vi "Puzzle 1-2.vi"() -> ()   [LabVIEW 2022 SP3]
panel:
  out "sum":i32=54265
  out "Array 3":i32[](array[numeric])=[91, 57, 81, 79, 28, 41, 41, 27, 45, 61, 17, 82, 27, 72, 45, 76, 32, 22, 13, 88, 15, 67, 85, 75, 55, 25, 75, 76, 72, 41, 58, 51, 13, 82, 73, 22, 73, 86, 32, 71, 92, 15, 49, 91, 17, 18, 32, 99, 77, 92, 38, 53, 25, 97, 22, 28, 84, 65, 28, 94, 47, 68, 63, 36, 66, 71, 51, 35, 91, 54, 43, 44, 18, 71, 96, 21, 37, 17, 27, 86, 38, 96, 16, 23, 51, 44, 72, 55, 71, 97, 82, 79, 99, 62, 88, 11, 88, 71, 65, 42, 61, 53, 33, 61, 39, 23, 24, 96, 24, 19, 65, 48, 11, 79, 38, 13, 13, 48, 21, 77, 55, 39, 32, 22, 16, 22, 64, 95, 96, 43, 29, 71, 22, 89, 29, 18, 91, 98, 43, 65, 11, 74, 63, 11, 74, 56, 41, 82, 38, 18, 71, 64, 96, 19, 81, 99, 13, 88, 95, 43, 15, 33, 46, 22, 87, 52, 29, 69, 92, 11, 17, 11, 96, 22, 96, 34, 32, 54, 43, 79, 56, 88, 51, 91, 71, 91, 37, 35, 66, 87, 71, 16, 14, 25, 16, 66, 98, 29, 31, 98, 87, 33, 18, 63, 62, 11, 88, 56, 66, 92, 18, 26, 94, 62, 58, 42, 19, 41, 64, 61, 52, 17, 92, 38, 79, 19, 95, 32, 35, 15, 96, 89, 67, 57, 53, 13, 36, 48, 89, 38, 71, 55, 55, 21, 85, 17, 55, 23, 28, 87, 77, 34, 39, 92, 19, 94, 72, 27, 37, 21, 22, 73, 57, 29, 42, 73, 64, 85, 64, 21, 72, 31, 54, 82, 65, 11, 22, 53, 28, 12, 94, 12, 62, 96, 47, 31, 74, 37, 33, 84, 42, 77, 28, 17, 34, 47, 42, 87, 36, 74, 98, 38, 49, 26, 28, 14, 23, 59, 88, 11, 15, 45, 85, 53, 19, 37, 86, 14, 52, 64, 48, 85, 71, 79, 11, 11, 79, 89, 89, 31, 56, 48, 95, 75, 63, 72, 89, 88, 58, 78, 47, 42, 15, 48, 77, 36, 85, 68, 93, 73, 52, 82, 58, 34, 22, 12, 86, 35, 91, 19, 13, 44, 95, 52, 58, 51, 65, 13, 61, 13, 87, 69, 63, 45, 24, 47, 42, 49, 28, 61, 21, 33, 99, 27, 65, 24, 74, 73, 74, 72, 29, 87, 94, 29, 88, 53, 24, 77, 45, 33, 64, 89, 16, 68, 92, 36, 98, 16, 78, 53, 27, 26, 34, 47, 88, 49, 23, 52, 88, 91, 99, 87, 62, 66, 88, 67, 57, 59, 61, 48, 69, 57, 55, 99, 22, 26, 45, 17, 63, 38, 74, 23, 17, 93, 63, 23, 91, 94, 54, 67, 55, 89, 57, 67, 89, 79, 29, 31, 48, 73, 48, 29, 17, 51, 44, 82, 72, 53, 12, 21, 11, 33, 56, 61, 53, 32, 98, 59, 66, 86, 46, 14, 89, 14, 11, 29, 79, 95, 67, 76, 88, 99, 42, 49, 53, 18, 35, 19, 33, 75, 64, 77, 24, 97, 41, 83, 94, 23, 99, 15, 24, 61, 72, 63, 44, 72, 13, 25, 64, 43, 28, 44, 37, 27, 53, 91, 95, 75, 66, 61, 38, 38, 54, 87, 96, 71, 29, 25, 81, 13, 11, 58, 74, 38, 32, 96, 35, 88, 34, 63, 75, 61, 41, 11, 11, 91, 39, 56, 77, 77, 77, 23, 87, 89, 17, 47, 55, 98, 52, 27, 91, 98, 87, 67, 35, 35, 15, 78, 19, 85, 17, 41, 23, 52, 97, 19, 68, 39, 43, 44, 27, 12, 86, 23, 87, 28, 49, 83, 92, 62, 72, 24, 23, 56, 18, 58, 32, 17, 11, 15, 77, 33, 84, 47, 73, 95, 82, 48, 43, 97, 35, 12, 13, 95, 27, 57, 67, 34, 88, 33, 99, 39, 97, 33, 62, 76, 63, 14, 84, 71, 52, 21, 37, 93, 48, 57, 29, 73, 14, 68, 19, 33, 97, 29, 86, 22, 92, 64, 42, 27, 66, 62, 22, 43, 68, 82, 44, 95, 74, 75, 37, 15, 89, 81, 43, 61, 53, 34, 45, 86, 31, 55, 43, 92, 88, 94, 87, 54, 41, 34, 45, 22, 63, 44, 23, 47, 54, 97, 18, 14, 77, 36, 48, 89, 49, 97, 71, 73, 41, 83, 91, 48, 89, 39, 97, 88, 28, 73, 61, 11, 62, 12, 24, 76, 22, 96, 18, 95, 56, 55, 17, 98, 61, 78, 73, 45, 94, 16, 65, 15, 88, 62, 57, 55, 91, 28, 99, 31, 61, 27, 79, 34, 64, 99, 42, 22, 13, 66, 37, 28, 22, 45, 65, 36, 77, 84, 14, 11, 29, 64, 97, 45, 96, 65, 18, 84, 29, 87, 32, 75, 89, 33, 17, 11, 39, 56, 79, 42, 75, 49, 72, 93, 39, 58, 16, 19, 36, 65, 44, 64, 52, 24, 16, 38, 74, 59, 38, 56, 65, 73, 72, 24, 27, 23, 11, 26, 82, 92, 82, 88, 79, 98, 44, 78, 91, 35, 14, 59, 58, 77, 98, 95, 95, 51, 15, 64, 46, 64, 38, 24, 85, 59, 17, 15, 62, 95, 22, 88, 14, 12, 52, 82, 22, 52, 83, 46, 55, 52, 22, 83, 54, 68, 53, 31, 26, 55, 35, 38, 58, 24, 33, 85, 81, 95, 32, 83, 54, 71, 71, 65, 45, 74, 96, 88, 33, 39, 14, 14, 71, 96, 43, 18, 56, 16, 66, 79, 23, 15, 54, 17, 85, 97, 23, 65, 94, 97, 59, 24, 66, 49, 31, 19, 19, 49, 66, 82, 75, 18, 86, 66, 98, 24, 44, 63, 63, 46, 33, 36, 97, 24, 47, 83, 74, 52, 95, 83, 52, 74, 11, 54, 49, 63, 88, 71, 54, 29, 55, 98, 56, 31, 48, 32, 71, 68, 11, 69, 86, 96, 49, 25, 33, 51, 91, 52, 48, 34, 37, 55, 48, 81, 48, 43, 69, 44, 49, 64, 94, 67, 99, 58, 86, 72, 78, 87, 46, 53, 27, 66, 89, 51, 42, 68, 47, 32, 57, 43, 72, 97, 87, 29]
  out "Array 2":string[](array[string])=["nine", "5", "8", "7", "2", "four", "four", "2", "4", "6", "1", "eight", "two", "seven", "4", "7", "3", "2", "1", "8", "1", "6", "eight", "7", "5", "two", "7", "7", "7", "4", "5", "five", "one", "8", "7", "2", "7", "8", "three", "7", "9", "1", "four", "nine", "1", "one", "three", "9", "7", "nine", "3", "5", "two", "nine", "2", "2", "eight", "six", "2", "nine", "four", "6", "six", "3", "6", "seven", "five", "3", "9", "5", "four", "4", "1", "seven", "9", "2", "three", "1", "2", "8", "three", "nine", "1", "2", "5", "4", "seven", "5", "7", "9", "8", "7", "9", "6", "eight", "1", "8", "seven", "six", "4", "6", "5", "3", "six", "3", "two", "two", "nine", "2", "one", "6", "4", "1", "7", "three", "1", "1", "4", "two", "7", "5", "three", "3", "2", "1", "2", "six", "nine", "9", "four", "two", "7", "2", "8", "2", "one", "nine", "9", "4", "6", "1", "seven", "six", "one", "7", "5", "4", "eight", "3", "1", "seven", "six", "nine", "one", "8", "9", "one", "eight", "nine", "four", "one", "3", "four", "2", "8", "five", "2", "6", "nine", "one", "one", "1", "nine", "2", "nine", "three", "3", "5", "4", "7", "5", "eight", "5", "nine", "seven", "nine", "three", "3", "six", "eight", "seven", "1", "one", "2", "one", "6", "nine", "two", "3", "9", "8", "3", "1", "6", "6", "one", "8", "five", "6", "nine", "1", "2", "9", "6", "5", "four", "1", "4", "6", "6", "five", "one", "9", "3", "7", "one", "9", "three", "3", "one", "nine", "8", "six", "five", "five", "1", "three", "4", "eight", "3", "7", "5", "five", "two", "eight", "one", "five", "two", "two", "8", "seven", "3", "3", "9", "one", "9", "seven", "two", "three", "2", "2", "seven", "5", "two", "4", "seven", "six", "8", "6", "2", "seven", "three", "5", "8", "six", "1", "two", "5", "2", "one", "9", "one", "six", "nine", "4", "3", "seven", "3", "3", "eight", "4", "seven", "2", "1", "three", "four", "four", "eight", "three", "7", "9", "3", "4", "two", "two", "one", "2", "five", "eight", "1", "one", "four", "8", "five", "1", "3", "8", "1", "5", "6", "four", "8", "7", "7", "1", "one", "seven", "8", "8", "3", "5", "4", "nine", "seven", "6", "seven", "eight", "8", "5", "7", "four", "four", "1", "4", "7", "three", "8", "six", "9", "seven", "five", "eight", "five", "three", "2", "one", "8", "three", "9", "one", "one", "four", "9", "five", "five", "5", "six", "1", "6", "one", "eight", "six", "6", "four", "2", "four", "4", "4", "two", "6", "two", "three", "9", "2", "six", "2", "seven", "7", "seven", "7", "two", "8", "nine", "two", "eight", "five", "2", "7", "four", "3", "six", "8", "one", "six", "9", "3", "9", "one", "seven", "5", "2", "2", "three", "4", "8", "four", "two", "5", "eight", "nine", "9", "eight", "six", "6", "eight", "6", "5", "five", "6", "four", "6", "5", "5", "9", "two", "two", "4", "1", "six", "three", "7", "2", "1", "9", "six", "2", "nine", "9", "five", "6", "five", "eight", "5", "six", "8", "7", "two", "3", "4", "seven", "four", "2", "1", "5", "four", "8", "7", "5", "1", "2", "one", "3", "five", "six", "5", "three", "9", "5", "6", "eight", "4", "1", "eight", "one", "one", "2", "seven", "9", "6", "7", "eight", "9", "four", "4", "5", "1", "3", "one", "3", "seven", "six", "7", "2", "9", "4", "eight", "9", "two", "9", "one", "2", "six", "7", "6", "4", "7", "1", "two", "six", "4", "2", "4", "three", "two", "five", "nine", "9", "7", "6", "six", "three", "three", "5", "8", "nine", "7", "two", "2", "8", "1", "1", "five", "seven", "three", "three", "nine", "3", "8", "3", "six", "seven", "6", "4", "one", "one", "nine", "3", "five", "7", "7", "7", "2", "8", "8", "one", "four", "5", "9", "5", "2", "nine", "9", "8", "6", "3", "3", "1", "seven", "1", "eight", "1", "4", "2", "5", "nine", "one", "6", "3", "4", "four", "two", "one", "eight", "2", "8", "2", "4", "eight", "nine", "six", "7", "two", "two", "5", "1", "5", "three", "1", "1", "1", "7", "3", "8", "four", "7", "9", "8", "4", "4", "nine", "3", "one", "one", "9", "two", "5", "6", "three", "8", "3", "9", "3", "nine", "three", "6", "7", "6", "one", "8", "seven", "5", "two", "three", "9", "4", "five", "two", "7", "one", "6", "1", "3", "9", "2", "8", "2", "9", "six", "four", "two", "6", "6", "2", "four", "6", "8", "4", "nine", "seven", "seven", "3", "1", "eight", "eight", "4", "6", "5", "3", "4", "8", "3", "5", "4", "9", "8", "9", "8", "5", "4", "three", "4", "2", "six", "4", "2", "4", "5", "9", "1", "one", "7", "3", "4", "8", "four", "9", "7", "7", "4", "8", "nine", "four", "eight", "three", "nine", "eight", "two", "7", "six", "1", "six", "one", "two", "seven", "2", "9", "one", "nine", "5", "5", "one", "9", "6", "7", "seven", "4", "nine", "1", "6", "one", "8", "6", "five", "5", "nine", "2", "9", "3", "6", "2", "7", "3", "6", "9", "4", "2", "one", "6", "3", "two", "2", "4", "6", "three", "seven", "8", "1", "one", "2", "six", "9", "four", "nine", "six", "1", "8", "2", "eight", "three", "seven", "8", "three", "one", "1", "3", "5", "7", "four", "7", "four", "seven", "nine", "3", "five", "1", "one", "3", "six", "4", "6", "5", "two", "one", "3", "seven", "5", "3", "5", "6", "7", "seven", "2", "2", "2", "1", "2", "eight", "nine", "eight", "eight", "seven", "9", "4", "7", "nine", "three", "1", "5", "five", "7", "9", "9", "nine", "five", "1", "six", "four", "6", "3", "two", "eight", "five", "1", "1", "6", "9", "2", "8", "1", "one", "5", "8", "two", "five", "eight", "four", "five", "five", "2", "8", "5", "6", "5", "3", "2", "5", "three", "3", "5", "two", "3", "8", "8", "9", "3", "eight", "five", "7", "seven", "six", "four", "7", "9", "eight", "three", "3", "one", "one", "seven", "9", "4", "one", "5", "one", "six", "7", "two", "one", "5", "1", "8", "nine", "2", "6", "nine", "9", "5", "two", "six", "four", "three", "one", "1", "4", "6", "eight", "7", "one", "8", "6", "nine", "2", "4", "6", "six", "4", "3", "three", "9", "2", "4", "8", "7", "5", "nine", "8", "5", "seven", "1", "5", "four", "six", "8", "seven", "5", "two", "five", "9", "five", "3", "four", "3", "7", "six", "one", "six", "eight", "nine", "4", "two", "3", "five", "9", "five", "four", "three", "three", "5", "4", "eight", "4", "four", "six", "4", "4", "6", "nine", "6", "9", "5", "eight", "seven", "seven", "eight", "4", "5", "two", "six", "eight", "5", "4", "6", "4", "three", "five", "4", "seven", "nine", "eight", "two"]
  out "Array":string[](array[string])=["1", "seven", "1", "9", "eight", "1", "1", "seven", "five", "one", "7", "two", "seven", "two", "5", "6", "2", "2", "3", "eight", "five", "seven", "five", "5", "5", "five", "5", "six", "two", "one", "eight", "1", "three", "two", "three", "two", "3", "6", "2", "1", "two", "5", "nine", "one", "seven", "eight", "two", "nine", "7", "2", "eight", "three", "5", "seven", "2", "eight", "4", "five", "8", "four", "seven", "eight", "three", "six", "6", "one", "one", "five", "1", "four", "3", "4", "eight", "1", "6", "one", "7", "seven", "7", "six", "8", "six", "6", "three", "one", "4", "2", "5", "1", "7", "two", "9", "9", "2", "eight", "1", "8", "one", "five", "two", "one", "3", "3", "1", "nine", "3", "four", "six", "four", "9", "5", "eight", "1", "nine", "8", "3", "3", "eight", "1", "7", "5", "nine", "2", "two", "six", "2", "4", "five", "6", "3", "9", "1", "2", "nine", "9", "8", "one", "8", "3", "5", "1", "4", "three", "one", "4", "six", "1", "two", "8", "eight", "1", "4", "six", "9", "one", "9", "3", "eight", "5", "3", "5", "3", "six", "2", "seven", "2", "9", "9", "two", "one", "seven", "1", "6", "2", "six", "4", "2", "4", "three", "nine", "6", "8", "1", "one", "1", "1", "7", "five", "six", "7", "1", "6", "4", "five", "6", "six", "8", "9", "1", "8", "seven", "3", "eight", "three", "2", "1", "eight", "six", "six", "2", "eight", "six", "4", "2", "8", "2", "9", "1", "four", "1", "two", "7", "2", "8", "nine", "nine", "5", "two", "5", "5", "six", "9", "7", "7", "three", "3", "6", "8", "nine", "eight", "1", "5", "5", "1", "five", "7", "5", "three", "eight", "7", "seven", "4", "nine", "two", "nine", "four", "two", "7", "7", "1", "2", "three", "seven", "nine", "2", "3", "4", "five", "4", "1", "two", "one", "four", "2", "five", "one", "2", "3", "8", "2", "4", "2", "two", "six", "7", "1", "four", "seven", "3", "four", "two", "7", "eight", "seven", "4", "7", "2", "seven", "6", "four", "eight", "eight", "9", "6", "eight", "four", "3", "9", "eight", "1", "5", "5", "5", "three", "nine", "seven", "6", "four", "2", "four", "8", "five", "one", "nine", "1", "one", "9", "9", "nine", "1", "six", "eight", "five", "5", "three", "2", "9", "8", "8", "8", "7", "2", "5", "eight", "7", "6", "5", "8", "3", "three", "2", "2", "eight", "4", "2", "2", "6", "five", "one", "9", "three", "4", "five", "2", "eight", "one", "five", "three", "1", "3", "7", "9", "three", "5", "four", "seven", "two", "9", "eight", "1", "1", "three", "9", "7", "5", "4", "4", "3", "four", "2", "nine", "seven", "4", "nine", "8", "3", "four", "7", "5", "three", "four", "9", "6", "8", "2", "six", "8", "6", "eight", "three", "7", "six", "four", "7", "8", "9", "3", "two", "8", "one", "nine", "7", "2", "6", "eight", "seven", "7", "9", "one", "eight", "nine", "seven", "5", "9", "two", "6", "five", "7", "3", "8", "4", "three", "seven", "3", "3", "3", "1", "four", "4", "seven", "5", "nine", "7", "7", "nine", "9", "9", "one", "eight", "3", "eight", "9", "7", "1", "4", "two", "two", "3", "two", "1", "1", "3", "6", "1", "three", "2", "8", "9", "6", "6", "six", "4", "nine", "4", "1", "9", "9", "five", "seven", "six", "8", "nine", "2", "nine", "3", "eight", "5", "nine", "3", "5", "4", "seven", "4", "7", "one", "3", "4", "3", "9", "five", "4", "one", "2", "3", "4", "2", "three", "5", "four", "three", "8", "4", "7", "7", "3", "one", "5", "5", "6", "one", "eight", "eight", "4", "seven", "6", "one", "9", "5", "1", "three", "1", "8", "4", "eight", "two", "six", "5", "8", "4", "3", "5", "1", "1", "1", "one", "one", "9", "6", "7", "7", "7", "three", "7", "9", "7", "7", "5", "8", "two", "seven", "one", "eight", "7", "seven", "5", "five", "5", "8", "nine", "5", "seven", "one", "3", "2", "seven", "9", "8", "nine", "three", "four", "7", "two", "six", "three", "seven", "eight", "nine", "3", "2", "two", "2", "four", "3", "6", "8", "eight", "two", "seven", "1", "5", "7", "3", "4", "7", "3", "five", "two", "8", "3", "seven", "five", "2", "three", "5", "7", "7", "7", "four", "eight", "3", "9", "nine", "seven", "3", "two", "six", "three", "four", "four", "one", "2", "1", "seven", "three", "8", "seven", "nine", "three", "4", "8", "9", "3", "seven", "9", "six", "2", "2", "4", "two", "7", "six", "two", "2", "3", "8", "two", "4", "5", "4", "five", "7", "5", "nine", "1", "three", "1", "3", "4", "5", "6", "one", "5", "three", "two", "8", "4", "seven", "four", "1", "4", "five", "2", "3", "4", "three", "seven", "4", "7", "8", "4", "seven", "6", "eight", "nine", "9", "seven", "1", "3", "1", "three", "one", "eight", "9", "nine", "seven", "8", "8", "three", "one", "1", "two", "2", "4", "six", "two", "6", "8", "five", "6", "five", "seven", "8", "one", "eight", "three", "5", "4", "6", "5", "five", "eight", "2", "7", "5", "1", "8", "9", "one", "one", "7", "nine", "four", "four", "9", "2", "2", "three", "6", "7", "eight", "2", "five", "five", "six", "seven", "4", "4", "1", "9", "four", "seven", "5", "6", "five", "8", "four", "nine", "seven", "2", "5", "9", "three", "7", "1", "nine", "6", "nine", "2", "five", "nine", "two", "three", "nine", "8", "6", "9", "6", "5", "four", "4", "two", "4", "6", "eight", "4", "9", "8", "6", "five", "three", "two", "4", "7", "three", "1", "6", "2", "2", "2", "8", "9", "eight", "4", "8", "one", "5", "four", "nine", "8", "7", "8", "five", "5", "1", "five", "four", "6", "four", "8", "four", "5", "9", "seven", "5", "two", "5", "2", "eight", "4", "2", "2", "2", "2", "two", "3", "6", "five", "two", "2", "three", "four", "8", "three", "one", "6", "five", "5", "eight", "eight", "four", "3", "5", "1", "5", "2", "three", "four", "1", "one", "five", "5", "4", "six", "8", "3", "9", "four", "four", "one", "6", "three", "8", "six", "6", "6", "nine", "3", "five", "4", "7", "5", "7", "3", "five", "4", "7", "nine", "four", "6", "nine", "one", "9", "nine", "9", "6", "2", "five", "8", "6", "six", "eight", "4", "4", "three", "3", "6", "three", "6", "seven", "four", "seven", "three", "four", "2", "five", "3", "two", "4", "1", "four", "9", "3", "8", "one", "four", "9", "5", "eight", "6", "1", "8", "2", "one", "8", "one", "9", "six", "6", "9", "5", "3", "1", "one", "two", "eight", "four", "7", "5", "eight", "one", "8", "three", "nine", "4", "nine", "four", "four", "7", "9", "8", "6", "two", "eight", "seven", "6", "three", "seven", "6", "9", "1", "2", "eight", "seven", "2", "seven", "3", "2", "7", "7", "9"]
  out "subarray":string[](array[string])=["ninefourone1", "53sevenvvqm", "kscpjfdxp895foureightckjjl1", "72fivebt9ndgq", "28gtbkszmrtmnineoneightmx", "four66jqrbtqcsxjtqjvfjhl1", "four8pzznjbhxlhtz6bhtzdxjlg1", "rgxjrsldrfmzq25szhbldzqhrhbjpkbjlsevenseven", "slkjvk4threesevenznjqmmfive", "61ppgrkmkfhteightone", "1threesix67px", "sxbjdbtlnjrmlzgxneightthreepmqxdxhfk8jfrheightwovp", "twofour2sevenk", "sevenonezknqnkfqbzffjvfivetwo94two", "45xj", "mp7one6eightvhfnmfive6", "fhtctftxm3threefour2b", "2dq7bdmhhs92", "pdnbqlbvtcxgpnfhmsfhzstgm173", "8fourvxkddsrlcvseveneight", "15zqpmsix77hlljgfive", "jzjv6seven", "eight1vbfive", "721sixsdzbqtskbpkqbcmgmlpk5psrhr", "pqxdxcx5", "twozsf2five", "7twosixthree775", "7xtxrch7six", "729twofourlqrxtwo", "qtvbgtclhnk4ninefourseven5one", "jvhngkcdjhnmqghdbqdzqssf5onegzjbbcchboneightn", "five8two14five2nine1", "one3twomddthree", "8nine9two", "7fiveeight9ninesix6fivethree", "254kcd61dc4two", "7sixonetxvthntlngtwobzkbz23", "8sixnine6", "threedqtgmv2skmvcd", "7ptdhpvr1", "lsvmzvzvd9mqxszjmbddkmxzdxsninedmglzlzphtwo", "kgdt12seven4xxtttr5", "nrdtgdftjmfour6fxjninenineblqlthvpcx", "ninezmstcdfchc11onebmmfdfhvdncrhc", "1fiveseven", "oneone26twoeight", "threefivenine98one9twotbbcq", "9cm7ninestc", "jcrbmcjtrlzvz7", "nine8nine22", "3nineoneseveneight", "58four2three", "stwonefourthree9twonine4six5bvxgkxf", "ninechzcz4seven", "2tgzgmtzzpjdqqz", "brsptjppb28qxcxxjbzpeighteight", "eightthree3ninejrft4", "sixqsgkzdjmgpfive4threemxltqdxsfive", "vxfd2q8", "khqhgqlxslkmbrvljcnineeight1gjgcqmnbdczqb8four", "mvbltrgpfourcclxftbb7gcbqcptvgfsevenrdm", "61eight", "six8fourthree6fourseven6three", "jqdfxvhjg3sflkn2sixptxxsqrfml", "6jtxs", "seven99threeone", "five6sevensmbbrjqvdbmkbsqtwonelg", "fdvfsndt32fourgllgfrninebhnzzczfive", "9hxp9srhjhjjvqljhzprcjpqreightzs1", "djldhkkcn55threethreefourflnxnbzhkzmx", "fourfive43chfvjnvjrkpxlgjrfnqbl", "fxjgtj4", "1sevenfour2fiveeight", "seven43rxxeightb1", "9sevensnxkp3lpzxfxnntkxzkrhk7jzhmtvn6", "25one", "threeone7", "1pkfvsxxthreeoneseven", "ztbvfqnpz2xdhgdjmgvfourtworqbxqsh47", "8four7sixninesix", "threedgl88cczqhqxjnc", "nineeightthree4sixfive3sixdqlmscqjk", "16crjsdl", "tgq2sixhc7three", "tzgsqspndt5xnqlthghzfvkkhone", "4fxdqrs64ninex34gd", "seven22", "kghfkrpvnppfncbhhqpt55bjf", "hjhb71bqdrrgsrkqdtsgrxgsscqjmtfzjkzsbp", "lgdnt9threeeighteight97", "pvjhnk83sixncvgmsjltwotdmmpxknhvntfndxr", "7449", "qdfzv9hkprplzkfh", "66three5five4zdsfrcnljqmsxf2", "veightwo27bdbsvseveneightrcqcjxsixeight", "1thvkkk", "8bnxqfsdhzppblzlzbkfsksfscmb", "zseventbdzlmhnnrfive1one", "sixxnmntrmp6srcsqbrqnjfiveeightfive", "4trnzlshnjtwo5twocxrvfssbj", "6two3twonetqt", "55qsnx43", "3three23tpctbkrnqv", "sixqk4cnfdmtltmlhqxtwo41glkhdhgnt", "35fivesevenpfournxzsbbgzthjvlvzrnine", "tworkzgkcvcone53nrvgdvgtc", "two9llkjbkz8pklrsgqqzr2four", "ninecgpbgcnine4tldjqsone4six", "2tfjhtfourfour", "onebhlhdvvqx1sevenmsixsix9", "pjgjt6jkrgshxltfnine8four45", "4vsqfljrfiveqeightnvbdb", "11nfslqvhm", "7crrhqxsfive8ctkzbhqnine", "vrvtglvthreettrkq5bdlrtpx718", "1btbxlthreedtrzgeightnineqczhqm3", "193", "fcbzxqxxjtmn47ffschdrbeight", "twoh1gqkrnm1", "7ninesixpzpsn7", "5kkvzpgqd", "three6nine", "32fdn", "22twoxgvktxpxmbjqtgtbckx", "1hdtftwosix", "2jfc", "six5nvzcgmrscjn5eight4", "nineqhtczsninetwosix4five", "9three6sj", "hntktlbqmldrphqzxkhfour193", "twotwo5259", "v7six1vtlxnpm", "rhsm2", "gprmtxbhlsv8onefournine", "2fsrbtdvft15six1kxpqbnqsxh9", "one5onemxthree8", "nineqbxdbznzktxsmstsntzffour3one", "9blhkhjsgsfgsblzdtqqfour8", "stz4889563cb", "vjrbs6threeptbbmncz7hqhqgfgldtseven5", "vbfs1", "zjqgczjsjpvzvjseven4", "sixfjzbrrhcfqvglxhnsxninedrvtvjbfqjdbrzblkq6three", "one3threegcdldjsrsssixonefiveonechngsl", "7srxv4hsgjqsqfvv1tdngkpjrczkl4", "5scgdglnjbnsix8fivesixtjccvmkfxfnzvhctgpncjc", "4eightfivefive1lgscbj7kpcr1", "eightknfssevenfive6jnpklczrpfeightwol", "37qccxllhzshninebvpc8", "1eightmmcthkhf", "seven8fourqn7tbgqnmzcc1", "sixsevenone4", "clhdvjnqnine9threesix", "onetwoeight9", "81z3threenjsdhnqxvtwonezv", "9hqtsb", "onekgnlbthreeg3", "eightspnrpjb65fivevzfpvjntbg7drbgjccneight", "ninerdlsix7285", "fournineninefive3vbnhmhdvjgdqcm", "njzspqxpxrone7four55", "nfdhlqcpvzrrtsmzhgq3", "fourmfdtnpsfbxkjtgtgx5sixrppsqplqdjvnsixdtqvtdm", "21onesix6sixnine2", "fffsmvtt8fivenineglrqrmktzzseven", "fivefoursevencjxmskrqclz2", "lgk27threefourfsqrbkntbkfourvflgrzhh9", "617hj9", "ninegcxninetwohpfdxrb3tjjjtxtnvtwo", "one1gnftc8onehtsxsmg", "foneight3fsbhdqzr5twojbsdnntwohd9seven", "zkzpfvcxqnbvrg1", "nine36cddqfvrf", "rdjlpfk2pschfsdrpz", "nine994three8six", "three3nvflpftf2eight4", "3nine2", "rxxjdk5354", "hf4eight8qjtcfldnkvtwofivetwothree", "7six3twodhnvmxj1nine", "57seven3six6", "qklbvzfhclfnllhhgeight8xtvld", "5fgzqhkssmkcfour1", "hhvjkdnlffnineeighttwo18twonecs", "sevenbfzrgfm1six1", "nine71cskklxvcbnxtskdbqnpgklrxklcgccxjnssksrlkx", "hmklhhjdthree77", "3vpxclbgkpone3ninesrclfive", "djfqkgjvqpfvdsix5sixtwoeightsix", "eightlt7csvgxpnslk", "sevenfoureightnld2mxtgpbzpthree1", "11sevenglfmsb6", "onetjjnxvssg1four4drxbxpnpv24", "2zdxs9mfnbgfmjln1threefive", "one186ltsbck", "6fsbpb9sixhc", "nine818", "xzqcpcdprsqjbgknkvztwo419q", "39qfdlcnkhg31", "9djnlcrxqxhrcb8mczrxrm", "nmb887525seven", "jhmv3", "zhvdbn1fivem8seven4sixoneighttsn", "6zmmjqmnftclqbcthree", "6cpzeight92", "onepqfhtsevencvlfvnczhb91mmtdprqxmcnine1", "tvqdfxn8eight", "five6fivercgrpbtjgv87jmcndclbk2six", "jgtmrbvl68lpqkpxddqqxvsixfivesix", "nine2nlffgkvmp", "1frdnhssftg4eightgclxsgqtn", "2sixblr94six", "94mlfv", "6vlqtcsmdd47hpfmlc7fiveeight2", "tklxghxv5bzc4hhcdcpmnine8", "four6one1zzgqghvs412", "xghjpblsfpg19ntpfmcfd", "471rbdblzs", "69fourhjxkvd7fourfour", "jmrscfqdfppfdjskpk61", "five5eightnqpd9ninezknztwo", "onelknchr7nrfprgmqzp", "svxlxrx9892five2", "3ntkbzzpxhdmrsix8ttgp", "ndh7zlnrzpvmnine", "one7xlnbmjjmfv62qvqjpfprbvjkpcnine", "99three5", "threetwotwo7dhtgtbchc7sixtwo", "tmfxxph3eightgdccscdsrkmnhbb75", "joneight4one5", "nine3six", "81tqzsqpkv99", "sixvjlq7", "five7bkc", "five3811threelfpzztxzk", "1fourkkpclqc3", "xgrpbmktcthree46g", "bgcp4two8", "jtgeightwo7nine", "bkmcrcq3eightrdtvrbglmxmmztqm", "7tscmg5one2jhhbfb1", "zt5khcrgqjg5nxxzxzd", "five85", "twothree1", "eightsixthreetwo6b3tnjmcqdjfive", "onefrlg7", "fivescbjxbdnvslqqsone5bdbvskpmksqmmfsncsmd", "two83fourthreefourseventhree", "dglrmbtkfltwofive8ninelzmrxvxoneeight", "8nine6sixsixtwo7", "sevennine4lbsevenkdnrhpltn", "h3fiveeight4cplrnd", "vhsgjbqm3ninedfhfsb", "93nine7jvjmlzgcztrqlxtwo", "zhhhdddbbgcssvfzdhmpone5fivefournine", "l9fourvjfbqpdslkmvxsdrnsgcvzpjxm", "kxlseven5two", "rbtwonegsdgvsjtpnnkone7mdz", "phffknvthree2threeqgvfqxgnine7", "2lgglnmthreeseven27three81", "lrgkrxx2", "seventwokxvzkvq6eightthree", "5fiveseven", "fstwonersngdlngx28nine", "49oneninesix8four2q", "hfvhzvmjgbfcbsevenrmhjhzkc3", "six84", "8eight2gzblldzvkjfive", "6fz3eightzmsqb4qsbbsnthm", "fcglpc2one51", "sevendqghclrpxt7pzone48two", "three5one", "5sevenfivebbzkjlcnxseven8fourmzqlxxgjvc", "xgg8one6782", "gggtljnnsix3lkhdqzzpdtdkmjtgjddkpgx4five", "qrmsfc13onevnhlbgs", "nrtwonethreerbbqffzh62", "5eight81gcdbrx3rlk", "mtdtxcmm2bgmqhgqrtxsn8", "onercx2", "9sixoneqgr4", "xmoneightfour2", "six85foursixninetwo", "ninetwo8four8six", "qchclfzq47", "khrll3two21", "seveneightnine8868four", "3rmbmtbxjp12seven", "3tsxgvqxmzvxbdvxtgrvdbzqbh", "eight7fourjtxx", "fmb4one7threekbxeightwoj", "vcsevensixseven577", "2dkhlrrtrnbgzrmxm5fiveclhgn1eight", "1sevenlmrbnfour17seven", "three5jtbvkseightoneseven4df", "fourrgqxplbpbxtsgkm7", "fourqdfxchlc371sc2", "fqxlmeighttwo1seven", "zvvlftlhfthreesix6three46qkstxvdt", "m74pjgccfour1four", "plphq933eighteight", "cdbqlhbhj3eight", "4onevgdkxhz799five9fbljhpqmvk", "two6qzgphxl", "two1eight", "onekxxghlonerqqlrs83threehvvdhsxmfour", "npmsvvrdl2673", "fivejthseightsixtwo9vgrvjzbzsrxjv", "eight2gqfive7mzjzpxqcvheightjfx", "1bxckdpt", "dngoneightbtdptfn85", "fourtwovfzgmxjseven935", "8onesix2drgjnlrxbtdlmlznine5", "five4mmpmqlttsx56ljdzldntdvthree", "1nxxgtwothree22twothreenine", "38eightsevennxctjfstp", "8fourvhnps3onellstpnztn6kvjccmv", "1bseven93eightfour", "5nphkdbhxqb2pqxtkvhxq", "nvvx6fourjgkdsczjv", "fourxrmq78", "8tjmnvthree3ninetwo2five", "p7cvtwoneq", "7thbggjbznrsixonethreeninej", "xdgm1crqfnklk", "onehmqqgh4ninenthjonegfjmvtfgd", "sevenbsqtlk9", "8seven9two9hdz29", "fbcjhzdgzdg8jgjvcrmgbcrsixnine", "3bssqrj44onedqxvhkfive1", "tmmxtz5dtxbbcjlfivesix", "pvfqzksgrs4khmlvtwoeightlsx", "psbttsmnpninefour42fivegsixfive", "sevenfiveqscr7dfxpninesix5", "xmsjddzfxftsjfq6four6eight6three", "seven42", "eighteight1nineeight9", "8c", "pmqljjjzvx5znxqnsfour8", "78zlpxnvsqpgmgmk", "four7fsgttnrgnlslr", "fourtwo3jg2", "qlz18three5lpxfjvnfppqjxh", "4fiveonetthree4eight", "7lzffxkxnzjrtr", "three7nineone46ksnshqgdpt", "8dntxkkkgdxggvhxh2onefour5gqzsqkm", "tjsixonedbklrxxk2twonxdpjzb8", "mfglbrjrq93", "seven37xhsrxrvcgninexbmdrzxthreeonethree", "fivegznvfztszqlhtrsslsmqq43212", "tdthjjjbkeighteightsevenpcbmpfq2", "five1eightq", "three13three4vrsrrtp", "cgztjgqgdths2", "dhxztfvlonetwokszrv8prdpm2", "dfkcklchjj8twonine52ppvndfcnf6", "three7ninenkxfourfive", "93sixlqxctdhmvssixone", "oneqbvfrvteightnineninefivethree9", "jskrtmvsrqnpvcgsmxbonecmlrjpdpc4three", "crpcfour54xxgzz", "9fivefhdpcqsd", "fivenineclfctjninefbsh2", "fivexhrzbqpfxl8sixtwoeightllzplcpllk", "zxgl5qneightsevenone", "sixpdc17thxfive", "1twolftpzbmnzvdlkvlsevenhdvgfrjhmthreethreeddkdvht", "67twotwo71", "oneeightcgnhtdxpfnsevenoneeight13", "eightthreervd5tnj17", "ssrsmhxrsixeight3gbqggcvfqg29", "6fivecvcdxnxhxxtlzthree", "fournrrsix595", "p2qchlvplzdvchkbdzzbnsix7ninefour", "fourthreefourtzvlrnr9m94seven", "4jxzkrfourvtjpsnrllkjcczmmqnsj4q1two", "4627qlpscgpjcnine539", "two6nineeight", "63five66fivethree1", "skndgzsbsntwoone1", "threerzgdxgtthree2three", "953lsdgn59", "27bk", "sixmfmbslpjjsixsvnqrvtxznffive5", "2ninenlgpggxm42six234", "fdzfvkjnchsevenfivethreetscllgjvrtqckfnmz3cszmt4", "7ninetlzsxjsl2nine3", "shsvptqngsevencjjthvfm9six5four", "7lsrq36threevzfjc62", "two59threedxmfourjfschvqvnine", "khfqjmksxhbvs8sevenhzrmjtkgm", "nine2stgflmsm8fkthhhjzlszdnmkmqpnjxrfc4", "twofourthree244nine", "eightvt978", "fivefiveninesixnine6513", "2lbtz19fourtshqsvblhrkhxbpfour", "ptt7bntxhdvl", "mskflsslvdlmndmmqmfourtczqlssnineseven5xxxkfvzd", "l329eightsevenfourfivethree", "rmlksxsixspp9fourhlcg", "8five9q", "hqoneightsix19nine6xmjbtgjzgrhmlrxq", "six38", "9eight2", "3sixbzhgfcg57sixsixjtqmknd", "9fchn58", "vrpftbnvonefour6", "vqgdtrvhnnxxsevenseven9eight", "56vnine5rdpsnlqcbq7three", "vncrjds2cmrg7", "213sixfivesix", "tzclpzdsthree4sxgjvrzcrzcndnfour", "4sixseven1three7", "8fbrggzmtqn8", "four79p", "twonineqonemfour3dq", "5fdgpmrghtksn5onesixtwo", "xseightwongqqsxtwo8jslclldvnb", "nine1one", "9gxjrfourvhqzcxdhrtpxgtwonine", "eighthfhtnvchtc7fjkrxsmhtm7rbk", "thqxcfjbksix32xqrgqsqtx", "6qjqql", "jgcreight7eight", "6onesix4threeseven", "5vcv1twoeight7", "fivesthreebvjntwo9jdxghmxvl", "632msc9threenineqfone", "dqxfourkb4eight", "6stsp3nine", "566sevenpdmg", "xprjdn55", "9mjtcmhjb", "twoninelkjznqztbc3twolnhjhdbfxmhfr", "twotczpxn6qlcfdlpnq", "4ninefive", "1rs44three2gzczjdgq7ssmtgjbgbb", "ggmzqbkgsix4five23bftjlmbfbd", "threehfcscmmlqvcjtpthree98", "7sixsixone4", "2fivefvrr9four4three", "1zt1seven", "9hsbthqvhhsnineone23tslqccg", "sixbqvd3", "22148four3", "ninejlpbtnfive41rtzqjgfmcbncrrlnn", "9sixfour", "qnhfivetwofjtqtlxd7lmrlfctq864", "69dqrzhlqssgcsxtz54cpmjvrkcfiveseven", "fiveqpv85frkmpgxgc", "xxqsscldeightone9ngqtkf1nine", "5sixgxbnnjsvhf5dgxgone7", "sixsevensqghlvkfxnfour7", "8gmgvjbfivesevennine", "qj796fourone9", "rmpfsppvzdtwo4threetwotwo9", "dqvtrhm3nhtrxxccmfiveonedfzfvcghr", "4threejxkhnxcxjoneightp", "sevenhkpfgdgsgnvseven3m", "qhrvjcnfdbqchrsvchcxfourbkhhq9six1eight", "29pqnd", "1oneonethree627", "5977rcr2threeeight1", "fournthpqbztrhnine64", "fjnjpgqxr86five4sixxhrtvbp2two", "7sdnvlb5two", "58vffgzcgx4nineoneeight3", "h1sjgqbhndbz1oneqgncmhnleightwos", "gjms21", "onetwodphfznine51", "gxpl3fourzfz3", "five46", "mqsixccffmc9gqk1", "5kvxpqrrpeightthree", "threefoursevenfive2dhtbrxlzzl", "shhczssbltllsmntntlqfqgnnl98rm", "5oneeight3vkqtwo29", "bv69fouronefourone6", "eight6five966", "4xnrtztgfgcmnmnsevensix", "gmsvtnjd1sevennine4xxhqfbrjjqbglqjngttc", "mdnxhhteightfive5onenineninegqjbqmfd", "xonefourtwo4", "onesix61", "sjmnjhkj2892eightnine9", "nzseven39", "99nnjjzdrfsnjhthree1sevenfive", "6xmggtbnblnbxdpkzblnvcvjqmhvntwoeightseven", "76five6six", "chdfjrlfhdzeight778", "xrvrck9five1hrvpfvkdcb7eightnine", "foureighttq5sgdfourl2", "4rnbxrhhboneonefournine", "5four3", "1b97eight", "hlcjghlhsf32tgknm565knxqr", "onecqgbgdcmlb2sixsix6nine", "kxdkz3", "seven5xvhrxdm", "xblqbgkqgsixvgrthreezxnzhknklxhbmgl4", "fvnkc7threethreeseven", "bmbqxv24jhdg", "97rfphlxvtx", "4pgblonelone", "ptdpllrddeight3", "9knpjzskrfd4", "twomjqdtbbvmj4shvsqrone3", "9zzh3pjsf6mhxlhm9glglfztjm", "cfconeight47fivetdsmndgvsmbqjvszb", "21vbqjz374", "sixeightqgfdjbhfd4oneeightone", "tbccqdpz78srmcdx4six2", "643gqtvhkljxt", "klfjf4qms", "zrnhkhqzpczzfqsgsrtxklpbtp72", "1cnqfltrmhphg832three", "twoseven5", "mxkmxlcgsixklclrkfr8638fourlrqpzgjq", "nkbfkh452pthree", "zvcktvd2485four88", "rfxj4", "three6jnr7", "two45rldjnmxkjphtwo7v", "fivelncjffdnkzqrshvthreeh3p", "ninejgrbmhrbqldeightnine6nine8one", "96lvpt2djrkc5", "7seveneightthcxgthreeseven5hpfddktpj", "6bvn", "sixbjxtphstzgspnmkcvc952one", "gmmslrndvltlthree394sevenoneightl", "threenine7onefourtwojxhzvqlseveneight", "5eightsix4txcczzmg", "84seven", "skjpkhxggsvjbprhllgjhninetwo6", "72bdpzccvone4zbdzlllnnonernlfvdpq", "bvrtmzmtwonine29", "mrlvmdnlxb2814five5fjxzlhpn", "lmrpf82rksix611", "tvq18oneqnmmzvtclnthree", "jrbjc1zbbpqbrddt26seven1", "lxfivenmdtnhdmf98ptpxsgmgrxkmmznlk", "zbmvchmxsevenddddthree2dxlddjp4", "three3onejg2fqgtjmpcgeighteight", "three2two9seightfjqtwo", "ninefive8sevenvnssix", "3cnbxxtgmf5", "kpmjcsfrjfgzhmbpnqmlvrhbhqs8", "3vvcone64", "fvqksdsixthreexbfivetwo3", "sevenseven5", "63twoone8vhbcpmmlfive1", "4ctwo17eightsixkpvlgpj1", "rsgsnone1", "kbvxonemcqfive3eightone", "ninenineone45threepvsmrtonejxmbnd", "37fklnjkslqk9th9", "fiveoneq8rcgdxtwo8jfkxq6", "rgd7", "7rgkdpvp7qrb", "7crtxfmslxxtcxsv", "mqdnltb23fiveqcdqtonethree", "8seven7", "8cqhqlhndqjznqhdbld2nspnxbj99tqqhp", "onelqn7", "bvbjfour7", "ldqzhvhrbgsrrkh5j", "kjsjxdcqgjztldjvxxgr9twoxfknxrrrphkdzdl8", "rvscnztblp56ljqtwompclcf", "2dbtdgsevenhzctckvkvxvjljz", "tvmhhxbbxvvsnlnineqsltjd92one", "9twoqdmtvbxhpcthreeeight", "81dvnkd87xbct", "6mnxqnndcjfivefdckzmppfsevenmqvvvbnrgs", "lvl3qjk5", "3fivefive", "ktvsqzrf14eightmtnqbcktk5", "sevencdknznbxseventwo8rzggmvpbvlrs", "hkhhrdxlml1xzbshninejzqc", "eightseven23shkgzdgvvcxxfdv5", "14five1sevenxfmhtptwo3seven", "47one", "2three3", "f5dszzs2", "xmxffxkxpkninethree8x6seven", "glzoneighteightrnjqgjznjm9", "63fznqxdfqt8", "33nine", "4vrbmthreefbdzf", "fourninethreesixnine9fourlvbgqhjbqncnlbjbz", "two848dbvbninenine17", "pqzqgone1two", "eight7lmxbhcsix", "szr2fcvkljctlghhthree", "sk81pxqhhhhvnjvgzfiveseven", "cgqqkrz2vpdpzrthqssg7nineeight", "498eightfournine", "eight85onesvxnineone53", "ninevmchpkcg2", "six2shsvqfivefourtwo", "mdzckfvr72cv", "twotwo7onethreefourdjtgjg", "tworfclmm3", "5sfvnkrmrptsix7four6kzlmclm", "1onedkqgzbr89kphvc8", "5seventhree8eight9eight", "kvjpgjgrcmpdscbfthreethree4mjqjnnzceightwohh", "kjbmh1fdkdtznmsznvlconeznineseven", "1fmgpxhxpqznqscvbszhhcmglvtnzhbbjjbzg", "1mfqzkfnine5", "rrflkqslxztdlqxqkdnhqd7ps", "39123thhsmscbpxr", "8vnine4jgqrvqtshg3jhhdnbsrxneight4", "xkqgnfour87", "lsbnjqtzqz7ninenineone73lmkbnkhs", "9fiveqqgqblfivehttxk", "8twotwognd", "4xknbheightfour6358", "4cqtpfjpf72eight3", "ninemjpqpqg8foureightsevenfcvpnrnnpzhcgkm", "37twofivedsxrzbpchnkgxqx", "oneone57one2k92", "mckoneight9threefour1onefourhdrcrvhqcmngkjnsthree", "945", "tmmtwo7", "57", "6twoxzbfftnr27", "threenine4bqpztsixfour", "84eight", "3jpbnjrqhqfnxckqkqdvls", "9gzzjzz", "374nine", "ninembxeight4sevent", "threecq3", "cvn6cvqmpmfflkzphndjnggtktwosn", "pgz7four5nineeightsixqrnfkdkgh", "6one781vstwothreef", "one617fourthreefourxqxnpv", "8eightsqmkjkkf5xckcvd4lfnnfour", "seven23qhntfmg56onexkjxh", "f5s56rfltx282", "twosixninefive1tlzq", "threetdhghclfsksql5oneninetwoseven", "zbqzxmpb9pxlrthree", "r4gxdzjnvzfonejnpmfcpgvxjjvkh8", "five338threejkk67seven", "twolntxcnzvfr55sixtwofivesevennine", "xhlppbqfr71brvppsixthreefddlgpfslqmdv", "kxsklgonefjfpkd4threefive9six4", "6srphqmtdoneh3glthreefour8", "rjzdmj1cqvxnx1nvcvbfctft9", "3fqjdgbpggthreesix53", "9fivesndgmkvckblktzkshglqgdl4ztwoseven", "qqrxkqhnzb23two34nine9", "8hrmffgstqpsixeightx1six", "jngcsjnrhn2zsvcjmjg", "9zfdmhzxdnfour272dcrqgk", "lbjbrfhjxhxjphzxsjsix4", "fourthree2seven1two", "twosix87", "vrlqqkctddggcvcjcpk6hxbqvbxmtsix", "mrcgbpc6dthzqmmthreefour6two", "r2zntjxgpfqfmqh", "fourseven3", "6nfnsgchjdffttmgfnbvlxzoneseven8", "8sevenqqfiveseven5twojvgk", "4rmtkvml4", "bprnine85", "sevenmfpcvlblcnine485fourseven4", "sevenseventhree68fivelhqgjqvcdqkvds", "3fourxsgghqnvtssnvfs7nine7", "1fiveone5hpfdgvxb", "eight2eight42twotwoonenine", "lpdeightxcgpxkkeighthtjpsninemjlxrxtg31", "4smqpjzsixonethree", "mr6csbmgrdrjj3onelqd4four1", "5sixvbscchd3", "384sps", "4qzgsvmfx4ninevcclvcfrfp6tckcpvj5s", "8l5glclltgcjgbhcg6", "3ldtdmjc6threeone", "hsrtzl521nine5qqrtpdsp", "z4v8threejdsmbfjpbj", "9sixln26eightwovmh", "848", "kndxtqpfrqxdxtfnqrqznpgvp9ninerlzcdvdtwo84", "kmqs84775seven", "5threefourzkg", "43five8cq2kprvdqrmxr1", "three4ttjqdh", "48nine7sixfive", "22x", "sixrgtwo3rnbzkrztkdkg", "4t", "29bjpskmxneightppvthree", "zmlzxvtlkt4seveneightbxseven", "5two5eightnpszzmbkncnstx4", "9vk98sevenhznkxmlrlk7vdbqgvfjdk", "1sixb8sjkvdhfld", "one42eight4mrsdnpfjpvdtq", "76fourntsrfllxkdfqvm6seven", "skqndhr3nm4776", "4xpmfxmvj633eight", "83ninecmpt", "fourdthree9", "9eightjqnnmthcrseven", "7threekgtf1", "xscj7threenmhsixseven5s3", "cqlzjt41", "855threemlmmqkgtfk", "ninefzmvjjtvbmgf8nineninetwonegcn", "ccpkzcldfourkdtfkjxvfb9fourhbtwonsoneightnl", "pkeightwo5seven88rdnzzsdkbjeight9", "threen2fjsfivesix26nine", "nine4rz8nine7bglpcmkqfzpseven", "eight94six8dpgrv", "twodfctf278", "fltqtmdkgjsvf72three", "llrtzsixsix4fivetwosixone", "qjhtjqjhgkjkzlpxxclsrdnzk1gbqt", "sixeight1sixtwo", "one5413nkmqjtlbdkz22", "bhtwoneonemzpzkqeighttwooneqkmcmsbq4", "sevensix3three2sixprcqcvm", "25tjffdrtwohfqlkhzxlhb", "97gcgqgjnpsthfjfdv636jsxq", "zggjmjone1297six8drzs", "jbpvnineeightntkkshbjvr3nshnqzdlkjmkfive", "5four2gkkbxmpthreefour6", "5two15sixfivetzpg", "one4fouronemfpvnqseven", "9fnlbljdnzzfournine78", "djfljccrtvvqktzzvk61onesd", "7twohbkeight", "seven1eighttwothreet", "4mdcljknhpqgxffqpj5", "nine9jlsmfgdgntwothreeeight4", "136nh", "635ninejghg5", "cmone7fdlk9lfivemzvnhkcsp", "8eightnlndm", "6fourpb892", "fiveseventwosixfourthree7", "5fm", "ninegchdnrf63431", "24sgnflnsixninenine8", "snm9", "3fntd721dhhkrqqxsfpstsvzpgonetkhcr", "jlzfbml61vdmgb7one", "266517", "7fivetwo2vhchmg678nine", "cgrp3vzn5ninetwofour", "666ninefour", "9s", "svpcnlktpxtvk42jhsvvdpftxpsk", "2qznfzvbdr", "foneb7eightfivehlbjjknninethree", "kfp6", "l34pxxhxtd7d", "rsbcrtwo27twocqlmeight", "jkzgvqgpjfdqvmjfx2flnvjmgllxghhrbjjkfour2", "45sevengdnf59twofive", "6fivespvkblrxvkcgdxktl", "three9dvrssvl5eight4ftsix", "seven56gdmlbfbjsl894sevencmc", "814", "1one4", "onenine5fivekcrf1gvvfhlncsv", "2ctvq9djzddfxcrj", "ntdlcqgsixvmfvlc4fourvlhtvvqmnmkrm", "9nineseven1seven", "lcvzbnfourksvjqvmv47one5", "nine4blvlvlpkl6", "sixnqxrhnztzvpmbzmxjm19five", "18jtzhk", "rzrhv8four", "2npghxvjonebchsprfhsjznrxvxnine", "eightngsevencrjkxbhpgtxlzhgb46sevenqhqmlfx", "threesffl9fivelgmndjfvseven92", "seven85", "87six9vnshclz", "threetwo7915three", "one2vkbp6rhqbxvcl7", "bsbr1five91", "qd3mnine", "jjvhltxtdh5nineone6", "mbxlnj7bbhnxonejtmtqjfrzqgtrhkeightnine", "fourfourqrxdtfive2smnqp", "7tvjrszvrhdl5five", "four15tvmpvxpvdjnine", "sevenvv5tworpvdlseven3dlqvgblqtwo", "nkckggninegnlqlnv25threexlhlbzvzk", "3vngmhprjseventhreeeightnine", "nvqtpzsszrdvttfivenine56oneseven8", "146", "fxfbone59", "f32dhffctkxp6rcngvtfq", "sixthreefsixjhckmjqfive495", "42four", "65nine984", "5fthreeone9twoqqsfvzmp", "ttwonefive4", "one6gfxseightxqcq6", "3sixnrjtwormrncmhxeight", "jhdxnmsgsdsevensqsslbsndpdmznmldbgeight3tcvjjv4", "5sixtvpckxzcjzbmrzk9", "pmdmnfgkb3six8xsmstsmxgmm", "53onetvlgbglq4zbqpdgsskzdsksd6", "kzjcllvz6skphkfdxfiveqrbhmk", "75qqjdgxlmfthreevzbfjdlxkfqqq", "seveneightjntpjthzptwo2two", "2five4fvrfxxnine4qzkkfkmq", "2xlvcltn7", "fnmggtj2rqxzh7three", "rzpjkgtml1", "2oneseven4one7xps6", "rljfhfrhmzkjxktnszbkpfspxdkqneight2", "pzgnine49six2", "plxsqeight2", "eight2sevenseveneight8rfcrsdlxb", "sevenclpqqfxgjnmtwo9", "9sevenrqsixone8eightrxqgfsbjh", "kqtkstrxhtfzbllhl4lqvqkcbr", "hfplfpbltczflpp7nfive8", "ninenvqfrvtwo6onel", "threev65", "frhn18six9sixninefourrsqzgd", "mcxckfg5vpkbs89gbninexjzvlj", "fivesixdx28", "7ppbqv", "hs9twopcvpgtjnrsvksskpc8", "9mlpckzj2twothreefive", "rkrgdclkninetwo6eighttwodc25", "tfivefourtwohkhhgsqlj1dtdcxmxkf", "1four6five", "fgbvmvxvtsix2twonine2sixfour", "foureight66", "s6fourcv", "mxl358sixfive8six8", "ztbtwo73sixvxsix9four", "eight7qmdlcxfive5", "phgfivekrjxdmnzsqsix9", "1mfqsevenhz", "rjhcdgzngtc155bqlttbsxklpknvlmk", "qjkdqlrrs6two", "sxlmqzxdpxdnj9fivetwo9seven5", "2qtdblb2", "8qgdzrsixtwo598oneightp", "1shdb944", "vrlpronek2", "jm52", "8eightfourseven11mvtrmtkr2bmp", "mnvnjxrgmrxhztwo2ssrdpqk", "ztfive435three6threetwo", "tnrrdnbgnbhzljdxhxxfrqkcpeight8js3", "foursix6zcsrztvgjxmp", "five7fourgnnkspxcmczcbgsbdf77five", "fgbrzkmvgrdbqjqndpfive81onetwomtzlfb", "2qbsfd1two3ninetwo2", "8tdjxvfpvdvone33three", "lpchnmln56twofive8tfour", "cfkfbhppjf6fourdkfxsvdtbcjspzlseven8", "5fivestgkzsevenonedkhhrkthree", "37nine8six8onefhvvbkmgdfgtv", "26hzz", "5glvnsztmnfjmkjseventdm4five", "pvnnqrqvftrbcvnnthreenine5", "mgscxxlp3eight", "53eighteight", "two1oneqlcdkbddfour", "jbll3", "8threeseven5tmtrgdhqxd", "8twonine6s1", "91seven5pmqrjlhqrtzs", "jj3sevensix4482", "jeightwo7lk4three", "zchchxmsctzffivefournine9sqhqkgfour", "72xct1", "vnsxvsqkhpfvgdseven23gzcmltzgone", "xzjqhcvsix1fivecjtxnfivekmvjdc", "zdfourgjlhtwo24d5klkpdgqbz", "7sdzzdbrxbtonerjcmknnql4dfzqccvqt", "tncqzxjq9twofiveqkxdrxrpj894six", "dddmkctrzlpfmsszeight8zvbpmpkg", "three23ckjhgjc", "375jzdhnfcfr19mhsbnplqh", "vpbbjlzone5sevenseven33four", "onejzfsevenrbskjq1four", "seven13one", "vcnkfgv979one6zln", "rqlxzzbmjb4lmbthreektqsdcfzbmdsfivethreenrxdlkqt", "qkoneight8", "5rfourfivenine94fdprsix", "onexonelzdh2lcbqpzq6", "six6v", "7gtgxqnnine", "tsljzhntwo3fourpbjncgmvf3fflvjxp", "vfkdone9fivecftvmjdk", "xc5three6eight94", "18363one7", "8fiveksshdlfmzhljhcmjrn7kpv5j", "xbhmxfhbjnjzmninethree7", "2933mkmdqjcl", "6ncvzqxfvgfive", "lnine5fivetb4qmfktnqjxs", "93187", "5mqninedzkfhbk", "two7eightntdbsix298four", "sixone3bspxqxggkmkrbcqrhfrxrlgjrlvfl96", "fourfivehqls3nine", "threedfklszn2threeqzhh7one", "mqmftzglone6kjpgglznhrjz89", "146cvkftscqsevensixnine", "nndhdgpd484hxdgjtfsdxxg9", "6mbzckbjphg", "eight6jbjtnld2mdjtd", "zjtzcqxb736five", "jlkdmone8", "gvjnjvmlfvcmvnfb8xcgjcmjqvz1bzcctvsixfzqjlhfkfk6", "vr6onejnjmrrldnsixsix5six", "ninembtmtkgbctlfive45cjzzrmgcscfbcgeight", "2mdvneightjzgffivefive4", "hmdnbxghxjxt4czshmsfzc", "61six18threehrcj", "six3five6eightkdfzhxcjkdhq3", "jrhqrqkpd4hsixdsbjdpscclmnnhknqq16", "jflzcxr3three", "threefourghvgsktkc93cmjmsgh8one6", "96fivesevenslklhsfmpz", "jgkpgfnnbq2pmspdfhsqxfour", "g4fourthreerpkdhjhlxlzvnineseven", "xkxhkphnkvpdnlncn86srxthree", "7sixsevenrfour", "5zr72qltsrbdsv", "ninervqzdfzqmf6five", "8jslpvs73", "ztvlxndlm5twohdhmtrdnhbzdrxb", "seven6nine4dpdpvrtrmqvql", "jfz1", "5nineeight5onefivecxtqbsdtbthreefour", "fourgeight6threeszgseventwo9", "sixfour3", "npl8", "tzjkffsvbjseven5rhmlxonezlx", "5dhtpfour", "twothreebxtfndvdnine1sixbb9", "five9nineqlzrmtgs5", "9v764nineeight", "five4eightlsix6", "3nineeight21", "foureight8btsc", "3xgdgtb2", "7threetwonexqk", "kkqsix48onefourhlsh8", "onekgtdzgfh2fivenine2onerb", "six4zgcnlhmltrxp5xphvtwo9", "eight7cdqggpssix", "niner9pzmrbqldkljmgphrrgmdjseven6", "439", "twofoursixrthree5bxppnhqtx", "bmpnt3", "fivepkzkzpghrptpksevenseven83two1", "9fiveone8one", "fiveseven3lqxghdlskbltrzrstwo", "fournine3ninephlghonetwoeightbvmdcconeightq", "three2pvklmzqjfh4sixonedrctlsfdfour", "three91spjlscscjcxbbpdhrg37", "57qqjpdfppsix1qxrh5mlmncf", "4nfone5eight", "eightqsix7one", "4jtvxfd38hnrmqkbnvfxpp", "qmfsspkfour1plmslcrsseventhree", "fzckcbfvxbpsix7nine", "fzrj4", "4threeqntnineqstzjftnine", "tkrh6sixdqflrvtmzmfiveseven9ktmtvprkxhfour", "nine4983four", "mpllmjrfgv66five3kvhthplrtwo7nkklb", "9ngvdjddqbz", "5twosix8lbhmzrg", "eightsbmcfgm76two4hhc6", "seventwosevenrpm6threeeightwodxs", "xkbseventwotwogmkxhpmhm42hvvbfchreight", "gcqeightwosix8xdlhrnnbkmsevenqdbrjghz", "458ninextfjxvgsq5fltdsk6", "rlgsflhxqd5bdbhclmrthree", "twothreemqqbzjn88blvqxbseven", "rqrrdrmlfsixfive6", "eight959tzxkgqjd", "txdszrn5eight3cqeight1brqr", "45122", "jvvslnkdk6qnfzjzvseight55eight", "4twoeightgrhhkrvtkrzpfive7seven", "three8gsmkpzsmfvf2", "fiveeight5sevenone9twoseven", "4seightjjdkdglspz3vg", "sevenssrzkspld2", "qnzcvcthrsgjlnzxmxlppjdpnine8seven7", "eight7xhvkrcr", "two2tdjdfbqtqxrs119r"]
  in  "delimited string":string="ninefourone1\n53sevenvvqm\nkscpjfdxp895foureightckjjl1\n72fivebt9ndgq\n28gtbkszmrtmnineoneightmx\nfour66jqrbtqcsxjtqjvfjhl1\nfour8pzznjbhxlhtz6bhtzdxjlg1\nrgxjrsldrfmzq25szhbldzqhrhbjpkbjlsevenseven\nslkjvk4threesevenznjqmmfive\n61ppgrkmkfhteightone\n1threesix67px\nsxbjdbtlnjrmlzgxneightthreepmqxdxhfk8jfrheightwovp\ntwofour2sevenk\nsevenonezknqnkfqbzffjvfivetwo94two\n45xj\nmp7one6eightvhfnmfive6\nfhtctftxm3threefour2b\n2dq7bdmhhs92\npdnbqlbvtcxgpnfhmsfhzstgm173\n8fourvxkddsrlcvseveneight\n15zqpmsix77hlljgfive\njzjv6seven\neight1vbfive\n721sixsdzbqtskbpkqbcmgmlpk5psrhr\npqxdxcx5\ntwozsf2five\n7twosixthree775\n7xtxrch7six..."
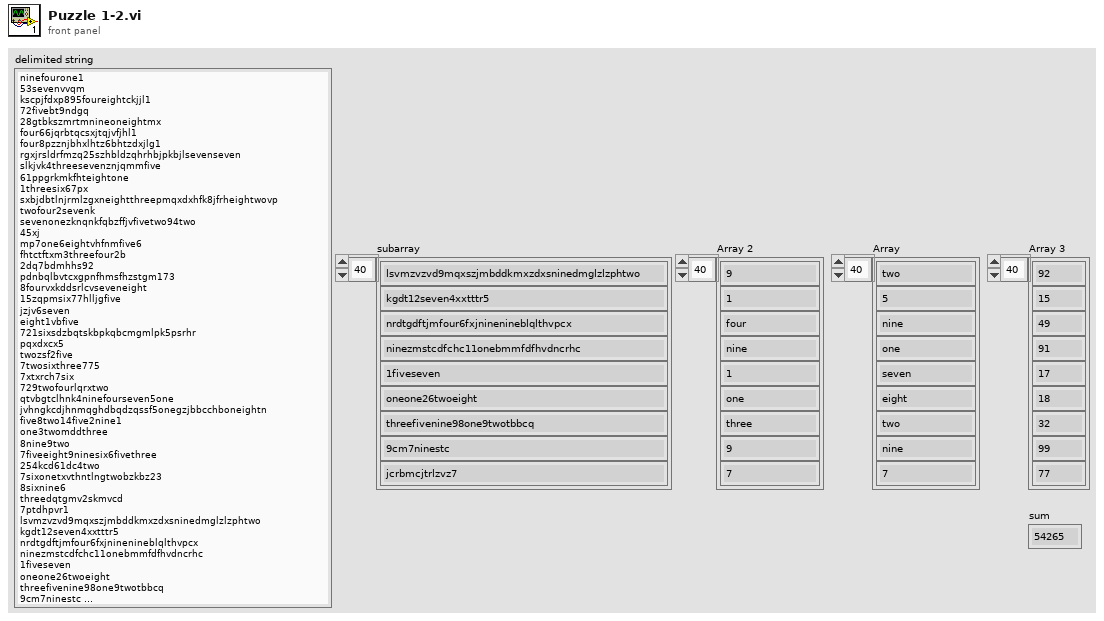
[diagram p1: front panel]
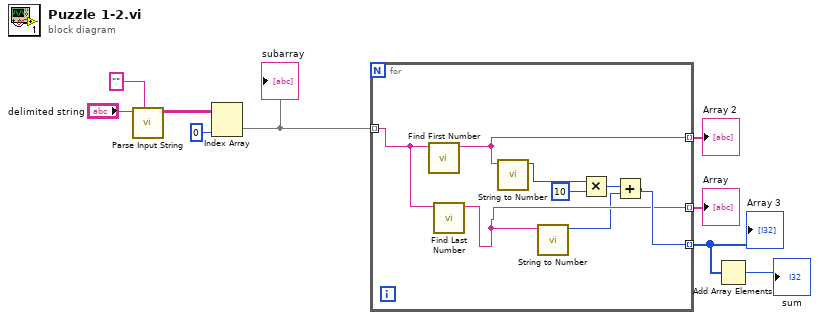
[diagram p0: block diagram]
diagram:
  n1 = call "Parse Input String.vi"("delimiter (Tab)"="", "delimited string"="delimited string") -> ("parsed string"=w7:string[][])  [unwired: 9 in]
  n2 = Index Array(array=w7, index (col)=0 ("disabled index (col)")) -> (element=w5:string[])  [unwired: 1 in]
  "subarray" <- w5
  n3 = for {
    tunnel: w5 -> [w14] mode=indexing
    tunnel: [w13] -> w4 mode=indexing
    tunnel: [w11] -> w3 mode=indexing
    tunnel: [w15] -> w2 mode=indexing
    n4 = call "Find First Number.vi"("String in"=w14) -> ("first number string"=w13:string)  [unwired: 10 in]
    n5 = call "Find Last Number.vi"("String in"=w14) -> ("first number"=w11:string)  [unwired: 10 in]
    n6 = call "String to Number.vi"("whole match"=w13) -> ("Numeric"=w12:i32)  [unwired: 10 in]
    n7 = call "String to Number.vi"("whole match"=w11) -> ("Numeric"=w10:i32)  [unwired: 10 in]
    n8 = Multiply(x=w12, y=10) -> (x*y=w16:i32)
    n9 = Add(x=w16, y=w10) -> (x+y=w15:i32)
  }
  "Array" <- w3
  "Array 2" <- w4
  "Array 3" <- w2
  n10 = Add Array Elements(numeric array=w2) -> (sum=→"sum":i32)
